vi "data type matches (not strict).vi"(8 "error in":errorcluster, 10 "Value":variant, 11 "data type":T1) -> (0 "error out":errorcluster, 3 "type match":bool)   [LabVIEW 2015, in "io runtime.lvclass"]
uses:
  io runtime.lvclass
  <vilib>/NI/Tag Bus/tag/Data Type.ctl
  <vilib>/Utility/VariantDataType/VariantType.lvlib
  <vilib>/NI/Tag Bus/tag/tag descriptor.lvclass
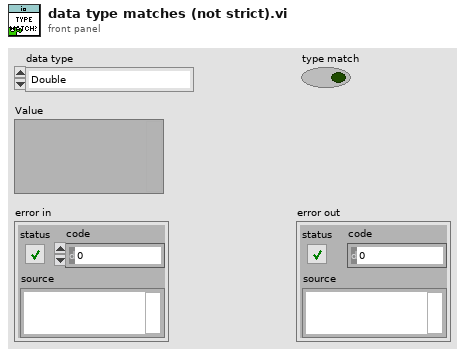
[diagram p1: front panel]
types:
  T1 = typedef "tag bus.lvlib/tag descriptor.lvclass/Data Type.ctl" = enum16{"Double", "Single", "I64", "I32", "I16", "I8", "U64", "U32", "U16", "U8", "Boolean", "String", "Array of Double", "Array of Single", "Array of I64", "Array of I32", "Array of I16", "Array of I8", "Array of U64", "Array of U32", "Array of U16", "Array of U8", "Array of Boolean", "Array of String"}
  T2 = typedef "VariantType.lvlib/Type.ctl" = enum8{"Invalid Type", "Void", "I8", "I16", "I32", "I64", "U8", "U16", "U32", "U64", "Single Float", "Double Float", "Extended Float", "Single Complex", "Double Complex", "Extended Complex", "Enum U8", "Enum U16", "Enum U32", "Enum U64", "Single Float With Unit", "Double Float With Unit", "Extended Float With Unit", "Single Complex with Unit", "Double Complex with Unit", "Extended Complex with Unit", "Boolean", "String", "Path", "Picture", "Tag", "Array", "Cluster", "Variant", "LV Variant", "Waveform", "Timestamp", "Digital Waveform", "Digital Data", "ExpressData", "Refnum", "External Data", "VI", "Poly VI", "LabVIEW Class Instance", "Fixed Point"}
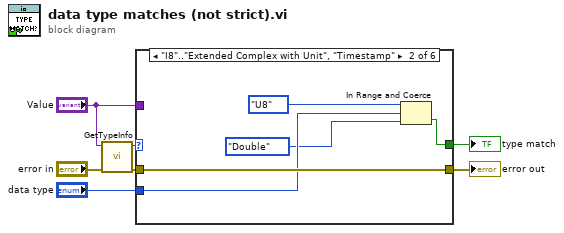
[diagram p0: block diagram]
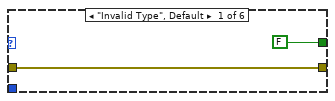
[diagram p2: hidden frame]
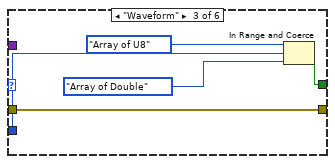
[diagram p3: hidden frame]
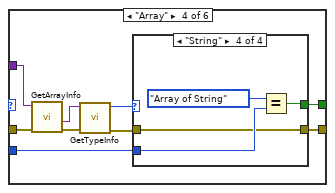
[diagram p4: hidden frame]
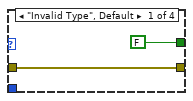
[diagram p5: hidden frame]
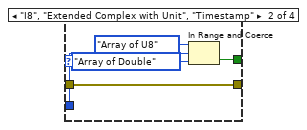
[diagram p6: hidden frame]
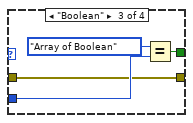
[diagram p7: hidden frame]
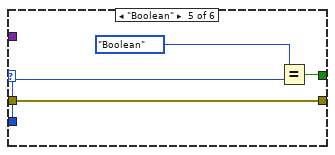
[diagram p8: hidden frame]
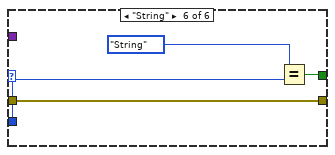
[diagram p9: hidden frame]
diagram:
  n1 = call <vilib>:"GetTypeInfo.vi"("error in (no error)"="error in", "Variant"="Value") -> ("error out"=w5:errorcluster, "Type Enum"=w4:T2)  [unwired: 5 in, 3 out]
  n2 = case shown="\"I8\"..\"Extended Complex with Unit\", \"Timestamp\"" w4 {
    tunnel: "Value" -> [_ _ _ w27 _ _]
    tunnel: w5 -> [w8 w14 w19 w28 w44 w48]
    tunnel: [FALSE w13 w18 w20 w47 w51] -> w6
    tunnel: "data type" -> [_ w12 w17 w25 w46 w50]
    tunnel: [w8 w14 w19 w26 w44 w48] -> w1
    frame "Invalid Type", Default {
    }
    frame "I8".."Extended Complex with Unit", "Timestamp" {
      n3 = In Range and Coerce(upper limit=Data_Type."U8", x=w12, lower limit=Data_Type."Double") -> (In Range?=w13:bool)  [unwired: 1 out]
    }
    frame "Waveform" {
      n4 = In Range and Coerce(upper limit=Data_Type."Array of U8", x=w17, lower limit=Data_Type."Array of Double") -> (In Range?=w18:bool)  [unwired: 1 out]
    }
    frame "Array" {
      n5 = call <vilib>:"GetArrayInfo.vi"("error in (no error)"=w28, "Variant"=w27) -> ("error out"=w24:errorcluster, "ArrayElement"=w23:variant)  [unwired: 6 in, 2 out]
      n6 = call <vilib>:"GetTypeInfo.vi"("error in (no error)"=w24, "Variant"=w23) -> ("error out"=w22:errorcluster, "Type Enum"=w21:T2)  [unwired: 5 in, 3 out]
      n7 = case shown="\"String\"" w21 {
        tunnel: w22 -> [w29 w35 w36 w40]
        tunnel: [FALSE w34 w39 w43] -> w20
        tunnel: w25 -> [_ w33 w38 w42]
        tunnel: [w29 w35 w36 w40] -> w26
        frame "Invalid Type", Default {
        }
        frame "I8", "Extended Complex with Unit", "Timestamp" {
          n8 = In Range and Coerce(upper limit=Data_Type."Array of U8", x=w33, lower limit=Data_Type."Array of Double") -> (In Range?=w34:bool)  [unwired: 1 out]
        }
        frame "Boolean" {
          n9 = Equal?(x=Data_Type."Array of Boolean", y=w38) -> (x = y?=w39:bool)
        }
        frame "String" {
          n10 = Equal?(x=Data_Type."Array of String", y=w42) -> (x = y?=w43:bool)
        }
      }
    }
    frame "Boolean" {
      n11 = Equal?(x=Data_Type."Boolean", y=w46) -> (x = y?=w47:bool)
    }
    frame "String" {
      n12 = Equal?(x=Data_Type."String", y=w50) -> (x = y?=w51:bool)
    }
  }
  "error out" <- w1
  "type match" <- w6
